vi "ReadDataFile.vi"() -> ()   [LabVIEW 2014]
panel:
  in  "Stringpath":string
  in  "Command":i32
  in  "Execute":bool
  out "Image Number":i32
  out "Events":u64
  out "Loop Count":i32
  out "data":u16[](array[numeric])
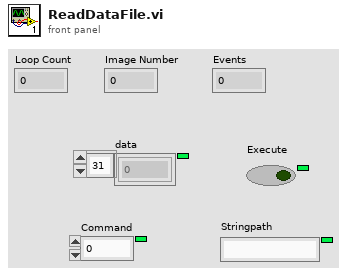
[diagram p1: front panel]
types:
  T1 = enum16{"big-endian, network order", "native, host order", "little-endian"}
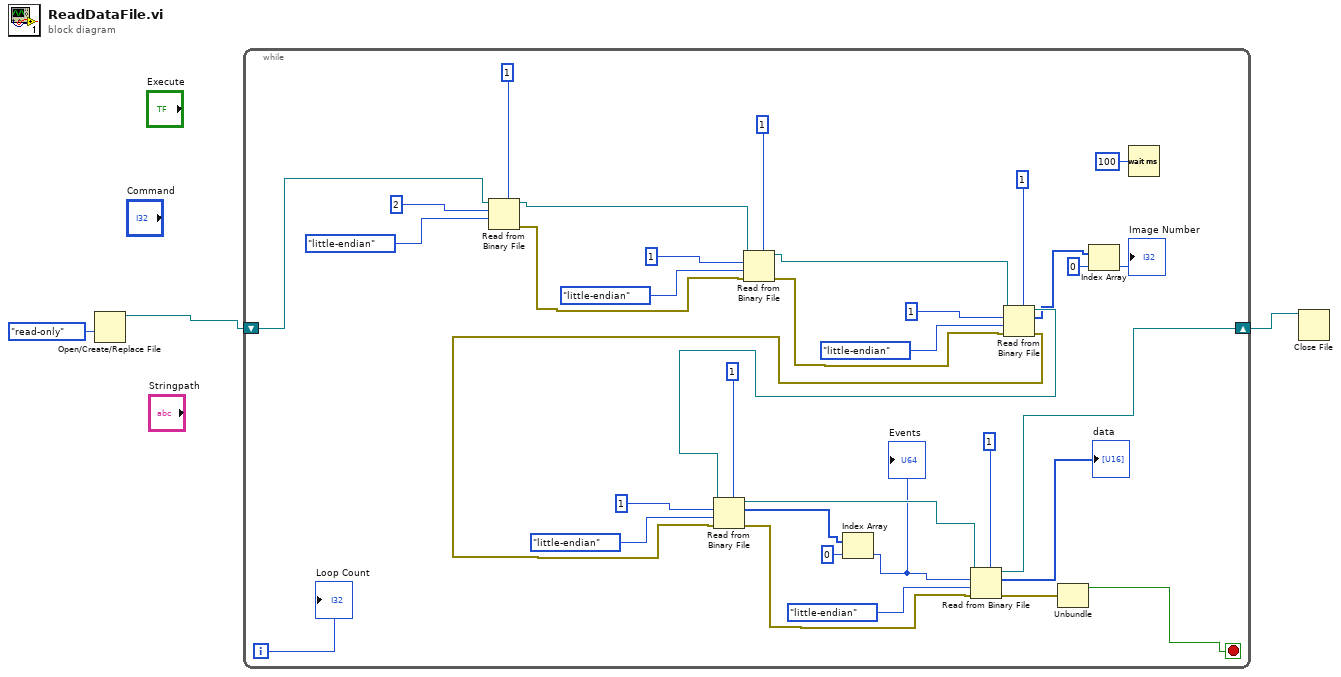
[diagram p0: block diagram]
diagram:
  n1 = Open/Create/Replace File(access (0:read/write)=enum16{"read/write", "read-only", "write-only"}."read-only") -> (refnum out=w3:refnum<file>)  [unwired: 5 in, 2 out]
  n2 = while {
    shift-right: [w10] -> w2
    shift-left: w3 -> [w9]
    i -> [w8]
    stop <- w11 stop-if-true
    n3 = Read from Binary File(5:1 ("count (1)"), 9:T1."little-endian" ("byte order (0:big-endian, network order)"), 10:2 ("count (1)"), 11:w9) -> (0:w31:errorcluster, 3:w32:refnum<file>)  [unwired: 2 in, 2 out]
    n4 = Read from Binary File(5:1 ("count (1)"), 8:w31, 9:T1."little-endian" ("byte order (0:big-endian, network order)"), 10:1 ("count (1)"), 11:w32) -> (0:w26:errorcluster, 3:w27:refnum<file>)  [unwired: 1 in, 2 out]
    n5 = Read from Binary File(5:1 ("count (1)"), 8:w26, 9:T1."little-endian" ("byte order (0:big-endian, network order)"), 10:1 ("count (1)"), 11:w27) -> (0:w22:errorcluster, 2:w5:i32[], 3:w21:refnum<file>)  [unwired: 1 in, 1 out]
    n6 = Read from Binary File(5:u64 1 ("count (1)"), 8:w22, 9:T1."little-endian" ("byte order (0:big-endian, network order)"), 10:1 ("count (1)"), 11:w21) -> (0:w18:errorcluster, 2:w16:u64[], 3:w17:refnum<file>)  [unwired: 1 in, 1 out]
    n7 = Index Array(array=w16, index=0) -> (element=w15:u64)
    "Events" <- w15
    n8 = Read from Binary File(5:u16 1 ("count (1)"), 8:w18, 9:T1."little-endian" ("byte order (0:big-endian, network order)"), 10:w15, 11:w17) -> (0:w13:errorcluster, 2:→"data":u16[], 3:w10:refnum<file>)  [unwired: 1 in, 1 out]
    n9 = Unbundle(w13) -> ("status"=w11:bool)  [unwired: 2 out]
    n10 = Index Array(array=w5, index=0) -> (element=→"Image Number":i32)
    n11 = Wait (ms)(milliseconds to wait=u32 100) -> ()  [unwired: 1 out]
    "Loop Count" <- w8
  }
  n12 = Close File(refnum=w2) -> ()  [unwired: 1 in, 2 out]
